vi "Settings.vi"(8 "error in (no error)":errorcluster, 9 "Gantry Region":i32=1, 11 "Syringe Space in":refnum<class "Syringe Space.lvclass">) -> (0 "error out":errorcluster, 3 "Syringe Space out":refnum<class "Syringe Space.lvclass">)   [LabVIEW 2019, in "Syringe Space.lvclass"]
uses:
  Syringe Space.lvclass
  C:/Users/HEP/Documents/Aerotech gantry/UCSB-Gantry-master/V5/Classes/Workspace/Fixture.lvclass
  C:/Users/HEP/Documents/Aerotech gantry/UCSB-Gantry-master/V5/Classes/Workspace/Carrier Tray/Assembly Tray.lvclass
  Fixture.lvclass/Fixture.ctl
  Assembly Tray.lvclass/Assembly Tray.ctl
  Write Fixture ID.vi
  Write Syringe.vi
  Write Gantry Region.vi
panel:
  in  "Submit":bool
  in  "Tray ID":i32=1
  # "Syringe Space"
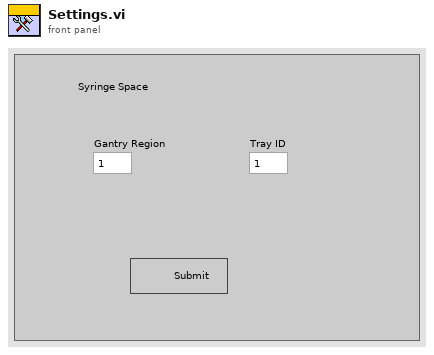
[diagram p1: front panel]
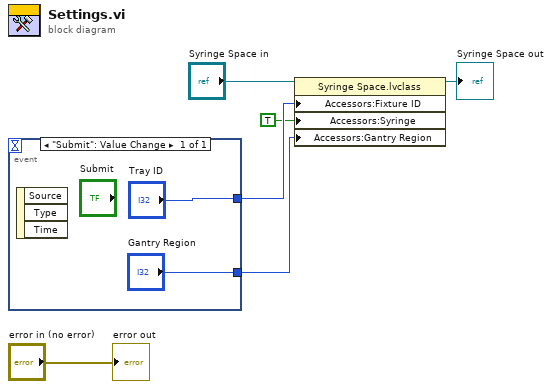
[diagram p0: block diagram]
diagram:
  n1 = event shown="[0] \"Submit\": Value Change" {
    selector: _ -> [_]
    dyn-events: _ -> [_]
    timeout: _ -> [_]
    tunnel: ["Tray ID"] -> w5
    tunnel: ["Gantry Region"] -> w2
    event "Submit": Value Change {
      n2 = event-data() -> ()  [unwired: 1 in, 3 out]
    }
  }
  n3 = property class="Syringe Space.lvclass"(reference="Syringe Space in", "Accessors:Fixture ID"=w5, "Accessors:Syringe"=TRUE ("Syringe"), "Accessors:Gantry Region"=w2) -> (reference out=→"Syringe Space out":refnum<class "Syringe Space.lvclass">)  [unwired: 1 in, 1 out]
  "error out" <- "error in (no error)"
